vi "move sub.vi"(0 "Pin 2 in":T1, 1 "Current position in":dbl, 2 "Set speed":dbl, 3 "mm to go":dbl, 5 "Pin 2 error in":errorcluster, 9 "Stepper 0 in":T1, 11 "Stepper 0 error in":errorcluster, 12 "Move":bool) -> (4 "Pin 2 out":T1, 6 "Pin 2 error out":errorcluster, 10 "Stepper 0 out":T1, 14 "Current position out":dbl, 15 "Stepper 0 error out":errorcluster)   [LabVIEW 2018]
uses:
  <vilib>/LabVIEW Interface for Arduino/Type Defs/Arduino Resource.ctl
  <vilib>/LabVIEW Interface for Arduino/Type Defs/Board Type.ctl
  <vilib>/LabVIEW Interface for Arduino/LabVIEW Interface for Arduino.lvlib
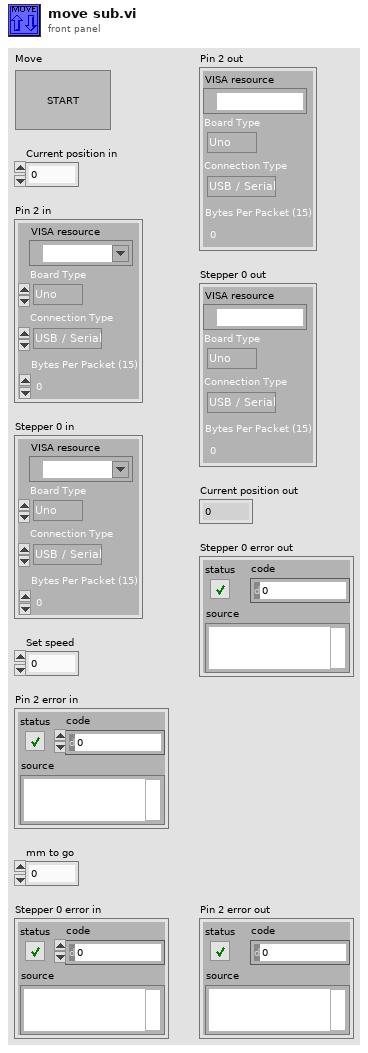
[diagram p1: front panel]
types:
  T1 = typedef "LabVIEW Interface for Arduino.lvlib/Arduino Resource.ctl" = cluster{"VISA resource":refnum<visa-resource-name>, "Board Type":T2, "Connection Type":enum8{"USB / Serial"}, "Bytes Per Packet (15)":u8}
  T2 = typedef "LabVIEW Interface for Arduino.lvlib/Board Type.ctl" = enum16{"Uno", "Dimuelanove w/Atmega 328", "Mega 2560"}
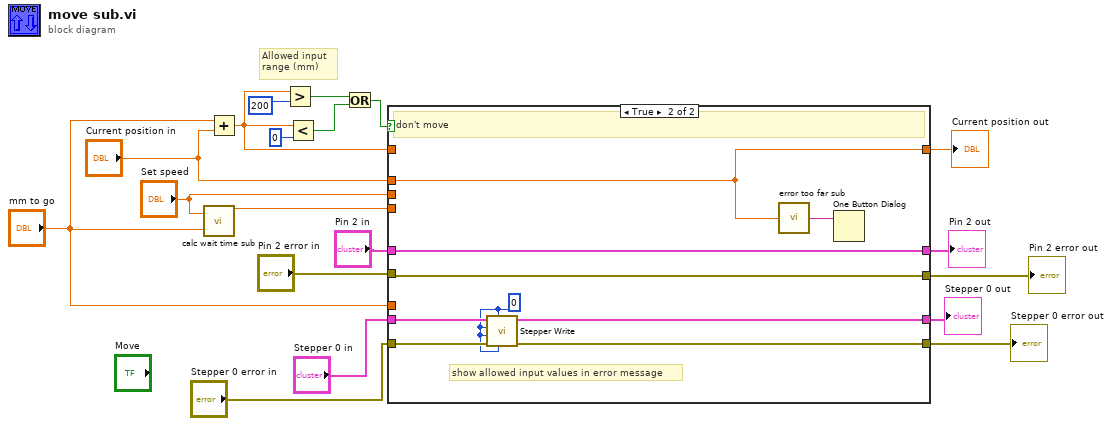
[diagram p0: block diagram]
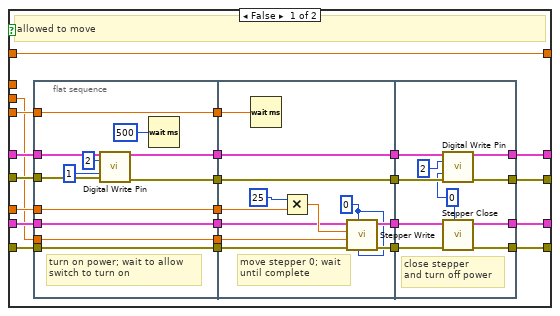
[diagram p2: hidden frame]
diagram:
  # "Allowed input\nrange (mm)"
  n1 = call "calc wait time sub.vi"("mm to go"="mm to go", "set speed (steps/s)"="Set speed") -> ("wait time"=w16:dbl)
  n2 = Add(x="mm to go", y="Current position in") -> (x+y=w4:dbl)
  n3 = Greater?(x=w4, y=200) -> (0:w10:bool)
  n4 = Less?(x=w4, y=0) -> (x < y?=w11:bool)
  n5 = Or(x=w10, y=w11) -> (x .or. y?=w1:bool)
  n6 = case shown="True" w1 {
    tunnel: [w33 w77] -> w7
    tunnel: [w36 w78] -> w8
    tunnel: "Stepper 0 in" -> [w40 w81]
    tunnel: "Stepper 0 error in" -> [w39 w80]
    tunnel: "Set speed" -> [w22 _]
    tunnel: w4 -> [w20 _]
    tunnel: "Pin 2 in" -> [w42 w84]
    tunnel: "Pin 2 error in" -> [w41 w83]
    tunnel: "mm to go" -> [w24 _]
    tunnel: [w28 w84] -> w15
    tunnel: [w27 w83] -> w19
    tunnel: w16 -> [w26 _]
    tunnel: [w20 w82] -> w17
    tunnel: "Current position in" -> [_ w82]
    frame False {
      # "allowed to move"
      n7 = flat-sequence {
        tunnel: w42 -> [w52]
        tunnel: w41 -> [w51]
        tunnel: w40 -> [w49]
        tunnel: w39 -> [w50]
        tunnel: [w50] -> w38
        tunnel: [w49] -> w37
        tunnel: [w48] -> w31
        tunnel: [w47] -> w29
        tunnel: w26 -> [w45]
        tunnel: [w45] -> w25
        tunnel: w24 -> [w44]
        tunnel: [w44] -> w23
        tunnel: w22 -> [w43]
        tunnel: [w43] -> w21
        tunnel: w38 -> [w65]
        tunnel: w37 -> [w64]
        tunnel: [w63] -> w35
        tunnel: [w62] -> w34
        tunnel: [w61] -> w32
        tunnel: w31 -> [w61]
        tunnel: [w60] -> w30
        tunnel: w29 -> [w60]
        tunnel: w25 -> [w59]
        tunnel: w23 -> [w56]
        tunnel: w21 -> [w58]
        tunnel: [w68] -> w36
        tunnel: w35 -> [w71]
        tunnel: [w69] -> w33
        tunnel: w34 -> [w70]
        tunnel: w32 -> [w75]
        tunnel: w30 -> [w74]
        tunnel: [w73] -> w28
        tunnel: [w72] -> w27
        frame #0 {
          # "turn on power; wait to allow \nswitch to turn on"
          n8 = call <vilib>:"Digital Write Pin.vi"("Arduino Resource"=w52, "Digital I/O Pin (0)"=2, "Value (0)"=1, "error in"=w51) -> ("Arduino Resource"=w48:T1, "error out"=w47:errorcluster)  [unwired: 10 in]
          n9 = Wait (ms)(milliseconds to wait=500) -> ()  [unwired: 1 out]
        }
        frame #1 {
          w55 = 0
          # "move stepper 0; wait\nuntil complete"
          n10 = Wait (ms)(milliseconds to wait=w59) -> ()  [unwired: 1 out]
          n11 = Multiply(x=25, y=w56) -> (x*y=w66:dbl)
          n12 = call <vilib>:"Stepper Write.vi"("Set Acceleration (0 to disable)"=w55, "Stepper #"=w55, "error in"=w65, "Set Speed (Steps per Second)"=w58, "# of Steps to Move"=w66, "Arduino Resource"=w64) -> ("error out"=w62:errorcluster, "Arduino Resource Out"=w63:T1)  [unwired: 4 in]
        }
        frame #2 {
          w67 = 0
          # "close stepper\nand turn off power"
          n13 = call <vilib>:"Digital Write Pin.vi"("Arduino Resource"=w75, "Digital I/O Pin (0)"=2, "Value (0)"=w67, "error in"=w74) -> ("Arduino Resource"=w73:T1, "error out"=w72:errorcluster)  [unwired: 10 in]
          n14 = call <vilib>:"Stepper Close.vi"("Stepper #"=w67, "error in"=w70, "Arduino Resource"=w71) -> ("error out"=w69:errorcluster, "Arduino Resource Out"=w68:T1)  [unwired: 7 in]
        }
      }
    }
    frame True {
      w79 = 0
      # "show allowed input values in error message"
      # "don't move"
      n15 = call <vilib>:"Stepper Write.vi"("Set Acceleration (0 to disable)"=w79, "Stepper #"=w79, "error in"=w80, "Set Speed (Steps per Second)"=w79, "# of Steps to Move"=w79, "Arduino Resource"=w81) -> ("error out"=w77:errorcluster, "Arduino Resource Out"=w78:T1)  [unwired: 4 in]
      n16 = call "error too far sub.vi"("current position"=w82) -> ("String"=w85:string)
      n17 = One Button Dialog(message=w85) -> ()  [unwired: 1 in, 1 out]
    }
  }
  "Pin 2 error out" <- w19
  "Current position out" <- w17
  "Pin 2 out" <- w15
  "Stepper 0 out" <- w8
  "Stepper 0 error out" <- w7
